vi "p1.vi"() -> ()   [LabVIEW 2023, in "d20.lvlib"]
uses:
  d20.lvlib
  Module Type.ctl
  AOC/AOC.lvlib
panel:
  out "Array":cluster{string, bool, string}[](array[cluster])
  in  "Example":string
  in  "Example":bool=TRUE
  out "Answer":u64
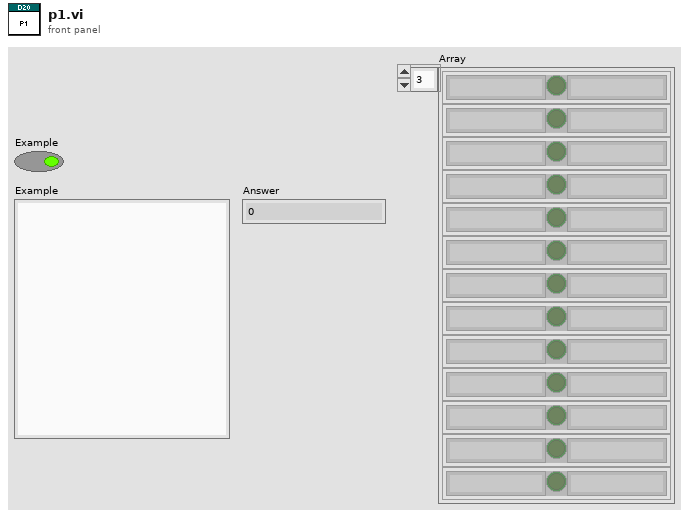
[diagram p1: front panel]
types:
  T1 = typedef "d20.lvlib/Module Type.ctl" = enum16{"broadcaster", "flip-flop", "conjunction", "output"}
  T2 = cluster{"Module Type":T1, "States":bool[], "string array":string[], "string array 2":string[]}
  T3 = map{string, cluster{"Module Type":T1, "States":bool[], "Destinations":string[], "Sources":string[]}}
  T4 = cluster{"Module Type":T1, "States":bool[], "string array":string[], "substring before match":string[]}
  T5 = cluster{"Module Type":T1, "States":bool[], "Destinations":string[], "Sources":string[]}
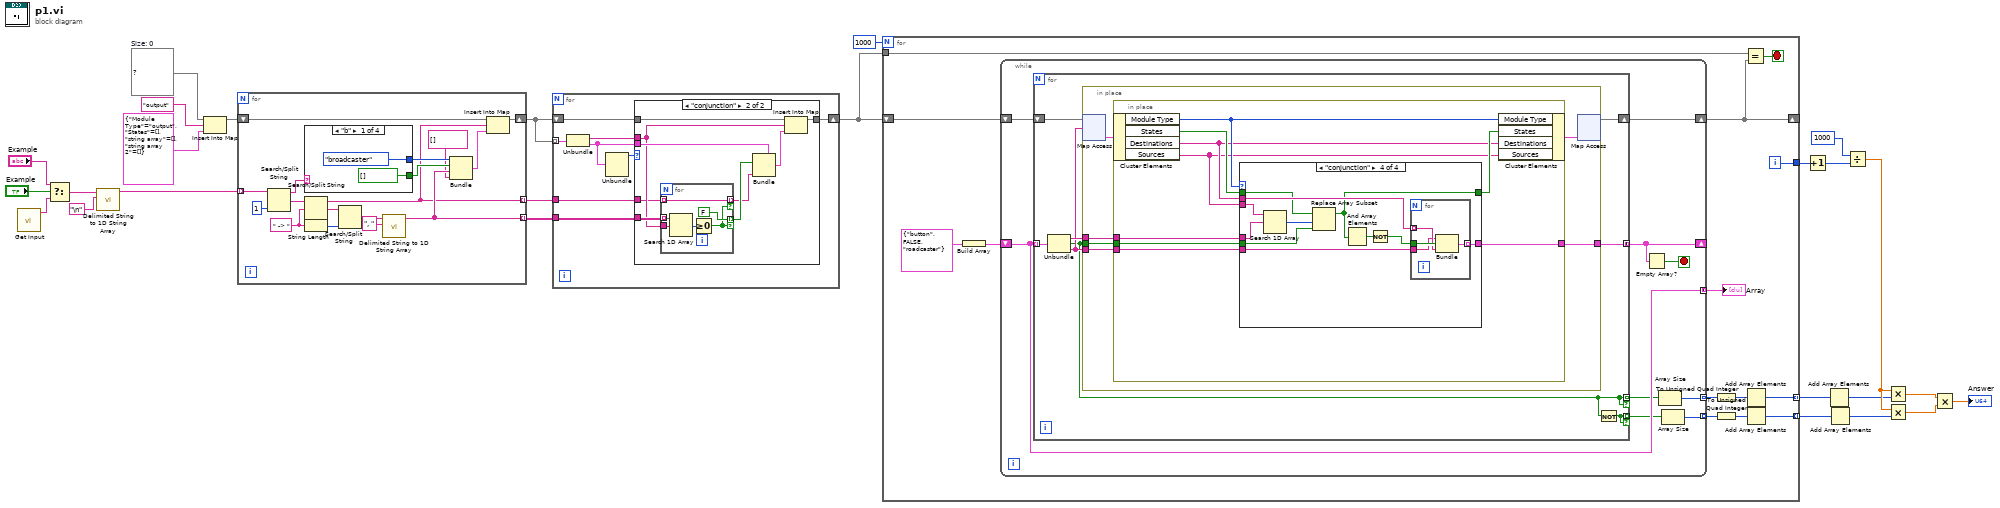
[diagram p0: block diagram]
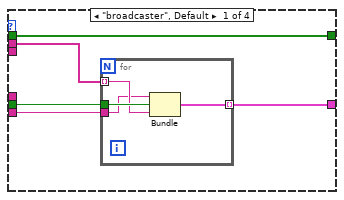
[diagram p2: hidden frame]
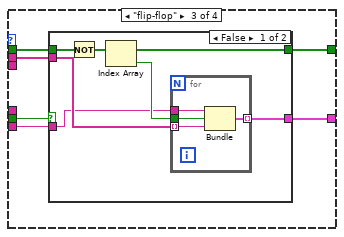
[diagram p4: hidden frame]
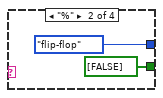
[diagram p7: hidden frame]
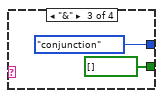
[diagram p8: hidden frame]
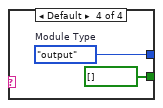
[diagram p9: hidden frame]
diagram:
  w20 = T3 {}  # Size: 0
  n1 = call "Get Input.vi"() -> ("Input"=w26:string)  [unwired: 11 in]
  n2 = Select(t="Example", s="Example", f=w26) -> (s? t:f=w23:string)
  n3 = call <vilib>:"Delimited String to 1D String Array.vi"("delimiter"="\n", "delimited string"=w23) -> ("string array"=w21:string[])  [unwired: 9 in]
  n4 = Insert Into Map(map in=w20, key="output", value=T2 {"Module Type"=enum."output", "States"=[], "string array"=[], "string array 2"=[]} ("output cluster")) -> (map out=w19:T3)  [unwired: 2 out]
  n5 = for {
    tunnel: w21 -> [w43] mode=indexing
    shift-right: [w40] -> w16
    shift-left: w19 -> [w39]
    tunnel: [w29] -> w15 mode=indexing
    tunnel: [w27] -> w14 mode=indexing
    w33 = " -> " ("search string/char (-)")
    n6 = Search/Split String(string=w43, offset (0)=1) -> (substring before match=w38:string, match + rest of string=w41:string)  [unwired: 1 in, 1 out]
    n7 = case shown="\"b\"" w38 {
      tunnel: [Module_Type."broadcaster" Module_Type."flip-flop" Module_Type."conjunction" w51] -> w37
      tunnel: [bool[] [] ("States") bool[] [FALSE] ("States") bool[] [] ("States") bool[] [] ("States")] -> w30
      frame "b" {
      }
      frame "%" {
      }
      frame "&" {
      }
      frame Default {
        w51 = Module_Type."output"  # Module Type
      }
    }
    n8 = Search/Split String(string=w41, search string/char (-)=w33) -> (substring before match=w27:string, match + rest of string=w35:string)  [unwired: 1 in, 1 out]
    n9 = String Length(string=w33) -> (length=w34:i32)
    n10 = Search/Split String(string=w35, offset (0)=w34) -> (match + rest of string=w32:string)  [unwired: 1 in, 2 out]
    n11 = call <vilib>:"Delimited String to 1D String Array.vi"("delimiter"=", ", "delimited string"=w32) -> ("string array"=w29:string[])  [unwired: 9 in]
    n12 = Bundle("Module Type"=w37, "States"=w30, "string array"=w29, "substring before match"=string[] []) -> (w36:T4)  [unwired: 1 in]
    n13 = Insert Into Map(map in=w39, key=w27, value=w36) -> (map out=w40:T3)  [unwired: 2 out]
  }
  n14 = for {
    shift-right: [w55] -> w13
    shift-left: w16 -> [w59]
    tunnel: w16 -> [w58] mode=indexing
    tunnel: w15 -> [w54]
    tunnel: w14 -> [w52]
    n15 = Unbundle(w58) -> (w57:string, "output cluster"=w53:T5)
    n16 = Unbundle(w53) -> ("Module Type"=w56:T1)  [unwired: 3 out]
    n17 = case shown="\"conjunction\"" w56 {
      tunnel: w59 -> [w60 w69]
      tunnel: w57 -> [_ w64]
      tunnel: [w60 w68] -> w55
      tunnel: w54 -> [_ w65]
      tunnel: w53 -> [_ w67]
      tunnel: w52 -> [_ w62]
      frame Default {
      }
      frame "conjunction" {
        n18 = for {
          tunnel: w65 -> [w73] mode=indexing
          tunnel: w64 -> [w72]
          tunnel: [FALSE] -> w63 mode=indexing if=w70
          tunnel: w62 -> [w71] mode=indexing
          tunnel: [w71] -> w61 mode=indexing if=w70
          n19 = Search 1D Array(1D array=w73, element=w72) -> (index of element=w74:i32)  [unwired: 1 in]
          n20 = Greater Or Equal To 0?(x=w74) -> (x >= 0?=w70:bool)
        }
        n21 = Bundle(cluster=w67, "States"=w63, "Sources"=w61) -> (w66:T5)  [unwired: 2 in]
        n22 = Insert Into Map(map in=w69, key=w64, value=w66) -> (map out=w68:T3)  [unwired: 2 out]
      }
    }
  }
  n23 = for {
    N: 1000 -> [_]
    tunnel: [w83] -> w9 mode=indexing
    shift-right: [w82] -> _
    shift-left: w13 -> [w89]
    tunnel: w13 -> [w81]
    tunnel: [w80] -> w12
    tunnel: [w77] -> w8 mode=indexing
    i -> [w80]
    stop <- w76 stop-if-true
    n24 = Build Array(cluster{string, bool, string} {"button", FALSE, "roadcaster"}) -> (w87:cluster{string, bool, string}[])
    n25 = while {
      shift-right: [w97] -> w82
      shift-left: w89 -> [w98]
      shift-right: [w94] -> _
      shift-left: w87 -> [w93]
      tunnel: [w96] -> w86 mode=indexing
      tunnel: [w93] -> w84 mode=concatenating
      tunnel: [w90] -> w79 mode=indexing
      stop <- w95 stop-if-true
      n26 = for {
        shift-right: [w103] -> w97
        shift-left: w98 -> [w106]
        tunnel: w93 -> [w105] mode=indexing
        tunnel: [w104] -> w94 mode=concatenating
        tunnel: [w100] -> w92 mode=indexing if=w100
        tunnel: [w99] -> w91 mode=indexing if=w99
        n27 = Unbundle(w105) -> (w102:string, w100:bool, w101:string)
        n28 = in-place {
          in-place-border: w100 -> [w112]
          in-place-border: [w111] -> w104
          in-place-border: w102 -> [w108]
          in-place-border: w101 -> [w107]
          n29 = in-place-map #1(w106, w101) -> (w110:T5)  [unwired: 1 in, 1 out]
          n30 = in-place {
            in-place-border: w112 -> [w121]
            in-place-border: [w120] -> w111
            in-place-border: w108 -> [w114]
            in-place-border: w107 -> [w113]
            n31 = in-place-cluster #2(w110) -> ("Module Type"=w118:T1, "States"=w119:bool[], "Destinations"=w116:string[], "Sources"=w115:string[])
            n32 = case shown="\"conjunction\"" w118 {
              tunnel: w121 -> [w126 _ w132 w150]
              tunnel: [w125 _ w134 w157] -> w120
              tunnel: w116 -> [w123 _ w136 w159]
              tunnel: w119 -> [w124 w131 w137 w153]
              tunnel: [w124 w131 w135 w152] -> w117
              tunnel: w115 -> [_ _ _ w155]
              tunnel: w114 -> [_ _ _ w154]
              tunnel: w113 -> [w122 _ w133 w156]
              frame "broadcaster", Default {
                n33 = for {
                  tunnel: w123 -> [w128] mode=indexing
                  tunnel: w126 -> [w130]
                  tunnel: [w129] -> w125 mode=indexing
                  tunnel: w122 -> [w127]
                  n34 = Bundle(w127, w130, "String"=w128) -> (w129:cluster{string, bool, "String":string})  [unwired: 1 in]
                }
              }
              frame "output" {
              }
              frame "flip-flop" {
                n35 = case shown="False" w132 {
                  tunnel: w137 -> [w143 w148]
                  tunnel: w136 -> [w142 _]
                  tunnel: [w141 w148] -> w135
                  tunnel: [w139 _] -> w134
                  tunnel: w133 -> [w138 _]
                  frame False {
                    n36 = Not(x=w143) -> (.not. x?=w141:bool[])
                    n37 = Index Array(array=w141) -> (element=w140:bool)  [unwired: 1 in]
                    n38 = for {
                      tunnel: w142 -> [w144] mode=indexing
                      tunnel: w140 -> [w147]
                      tunnel: [w146] -> w139 mode=indexing
                      tunnel: w138 -> [w145]
                      n39 = Bundle(w145, "Boolean"=w147, "String"=w144) -> (w146:cluster{string, "Boolean":bool, "String":string})  [unwired: 1 in]
                    }
                  }
                  frame True {
                  }
                }
              }
              frame "conjunction" {
                n40 = Search 1D Array(1D array=w155, element=w154) -> (index of element=w151:i32)  [unwired: 1 in]
                n41 = Replace Array Subset(array=w153, new element=w150, index=w151) -> (w152:bool[])
                n42 = And Array Elements(Boolean array=w152) -> (logical AND=w158:bool)
                n43 = Not(x=w158) -> (.not. x?=w149:bool)
                n44 = for {
                  tunnel: w159 -> [w161] mode=indexing
                  tunnel: w149 -> [w163]
                  tunnel: [w162] -> w157 mode=indexing
                  tunnel: w156 -> [w160]
                  n45 = Bundle(w160, w163, "String"=w161) -> (w162:cluster{string, bool, "String":string})  [unwired: 1 in]
                }
              }
            }
            n46 = in-place-cluster #2("Module Type"=w118, "States"=w117, "Destinations"=w116, "Sources"=w115) -> (w109:T5)
          }
          n47 = in-place-map #1(w109) -> (w103:T3)  [unwired: 1 in, 2 out]
        }
        n48 = Not(x=w100) -> (.not. x?=w99:bool)
      }
      n49 = Empty Array?(array=w94) -> (empty?=w95:bool)
      n50 = Array Size(array=w92) -> (size(s)=w96:i32)
      n51 = Array Size(array=w91) -> (size(s)=w90:i32)
    }
    "Array" <- w84
    n52 = To Unsigned Quad Integer(1:w86) -> (0:w85:u64[])
    n53 = To Unsigned Quad Integer(1:w79) -> (0:w78:u64[])
    n54 = Equal?(x=w81, y=w82) -> (x = y?=w76:bool)
    n55 = Add Array Elements(numeric array=w85) -> (sum=w83:u64)
    n56 = Add Array Elements(numeric array=w78) -> (sum=w77:u64)
  }
  n57 = Increment(x=w12) -> (x+1=w10:i32)
  n58 = Add Array Elements(numeric array=w9) -> (sum=w3:u64)
  n59 = Add Array Elements(numeric array=w8) -> (sum=w2:u64)
  n60 = Divide(x=1000, y=w10) -> (x/y=w7:dbl)
  n61 = Multiply(x=w7, y=w3) -> (x*y=w6:dbl)
  n62 = Multiply(x=w7, y=w2) -> (x*y=w5:dbl)
  n63 = Multiply(x=w6, y=w5) -> (x*y=→"Answer":dbl)
